vi "Manual Progress Bar Caller.vi"(7 "# of Steps":u8, 8 "Error In":errorcluster, 11 "Delay Label":string) -> (0 "Error Out":errorcluster)   [LabVIEW 2018]
uses:
  Misc/Global.vi
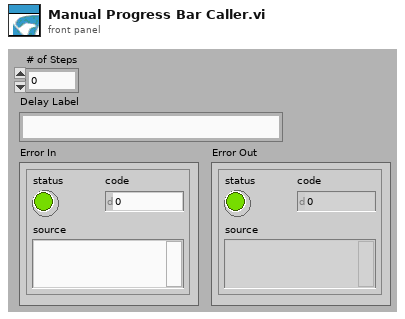
[diagram p1: front panel]
types:
  T1 = enum32{"Invalid", "Standard", "Closed", "Hidden", "Minimized", "Maximized"}
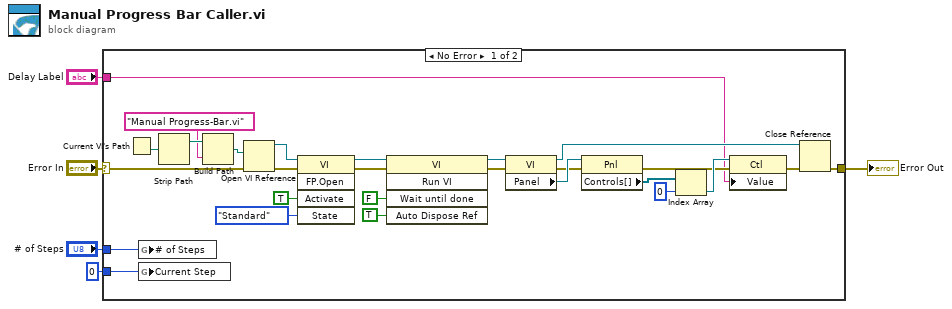
[diagram p0: block diagram]
diagram:
  n1 = case shown="No Error" "Error In" {
    selector: "Error In" -> [w17 w33]
    tunnel: "# of Steps" -> [w32 _]
    tunnel: [w20 w33] -> w4
    tunnel: "Delay Label" -> [w18 _]
    tunnel: u8 0 ("# of Steps") -> [w6 _]
    frame No Error {
      n2 = Current VI's Path() -> (path=w31:path)
      n3 = global write "Global.vi" "# of Steps"(w32) -> ()
      n4 = global write "Global.vi" "Current Step"(w6) -> ()
      n5 = Strip Path(path=w31) -> (stripped path=w30:path)  [unwired: 1 out]
      n6 = Build Path(base path=w30, name or relative path="Manual Progress-Bar.vi") -> (appended path=w28:path)
      n7 = Open VI Reference(vi path=w28, error in (no error)=w17) -> (vi reference=w15:refnum<vi>, error out=w16:errorcluster)  [unwired: 4 in]
      n8 = invoke class="VI" method="FP.Open"(reference=w15, error in=w16, "Activate"=TRUE ("Activate?"), "State"=T1."Standard") -> (reference out=w9:refnum<vi>, error out=w10:errorcluster)  [unwired: 1 in, 3 out]
      n9 = invoke class="VI" method="Run VI"(reference=w9, error in=w10, "Wait until done"=FALSE ("Wait Until Done"), "Auto Dispose Ref"=TRUE ("Auto Dispose Reference")) -> (reference out=w12:refnum<vi>, error out=w11:errorcluster)  [unwired: 1 in, 3 out]
      n10 = property class="VI"(reference=w12, error in=w11) -> (reference out=w21:refnum<vi>, error out=w22:errorcluster, "Panel"=w27:refnum<vi>)
      n11 = property class="Pnl"(reference=w27, error in=w22) -> (error out=w23:errorcluster, "Controls[]"=w26:refnum<vi>[])  [unwired: 1 out]
      n12 = Index Array(array=w26, index=0) -> (element=w24:refnum<vi>)
      n13 = property class="Ctl"(reference=w24, error in=w23, "Value"=w18) -> (error out=w19:errorcluster)  [unwired: 1 out]
      n14 = Close Reference(reference=w21, error in (no error)=w19) -> (error out=w20:errorcluster)
    }
    frame Error {
    }
  }
  "Error Out" <- w4
